vi "readCommandId.vi"(8 "error in (no error)":errorcluster, 10 "Parser":refnum<class "U8ArrayParserAutoIndexing.lvclass">, 11 "M1M3SAL in":refnum<class "M1M3SAL.lvclass">) -> (0 "error out":errorcluster, 2 "CommandId":variant, 3 "M1M3SAL out":refnum<class "M1M3SAL.lvclass">)   [LabVIEW 2016, in "M1M3SupportCommunicator.lvlib" / "M1M3SAL.lvclass"]
uses:
  M1M3SAL.lvclass
  Common_RT_Utilities/U8ArrayParserAutoIndexing/U8ArrayParserAutoIndexing.lvclass
  DataTypes/Topics/Parts/CommandId.ctl
  DataTypes/Topics/M1M3SupportTopics.lvlib
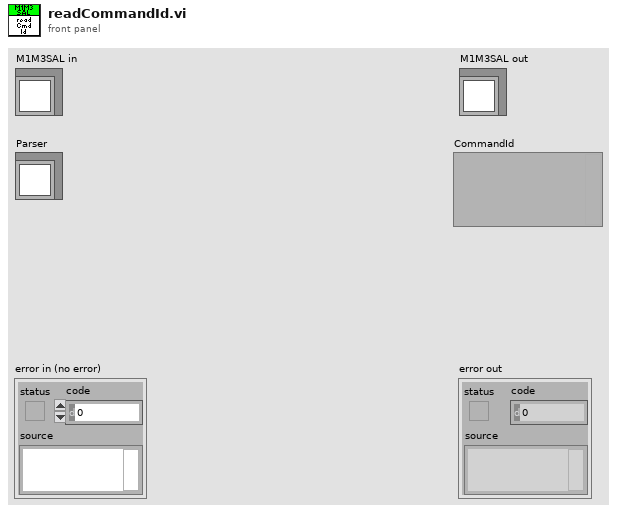
[diagram p1: front panel]
types:
  T1 = typedef "M1M3SupportTopics.lvlib/CommandId.ctl" = i32
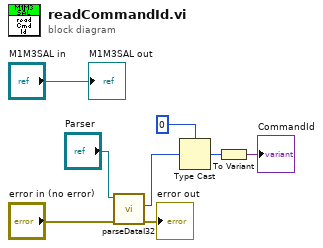
[diagram p0: block diagram]
diagram:
  n1 = call "parseDataI32.vi"("error in (no error)"="error in (no error)", "U8ArrayParserAutoIndexing in"="Parser") -> ("error out"=→"error out":errorcluster, "Data"=w3:i32)  [unwired: 7 in, 1 out]
  n2 = Type Cast(type=T1 0 ("CommandId"), x=w3) -> (*(type *) &x=w1:T1)
  n3 = To Variant(anything=w1) -> (Variant=→"CommandId":variant)
  "M1M3SAL out" <- "M1M3SAL in"
